vi "Build_Asylum_SetSTFC.vi"(6 "trigger":cluster{"Value":dbl, "greaterOrLesser":dbl}, 7 "eventString":string, 8 "error in (no error)":errorcluster, 9 "inChannelString":string, 10 "time":dbl, 11 "z":cluster{"Start":dbl, "End":dbl}) -> (0 "error out":errorcluster, 3 "Command":string)   [LabVIEW 2020]
panel:
  in  "callback":string
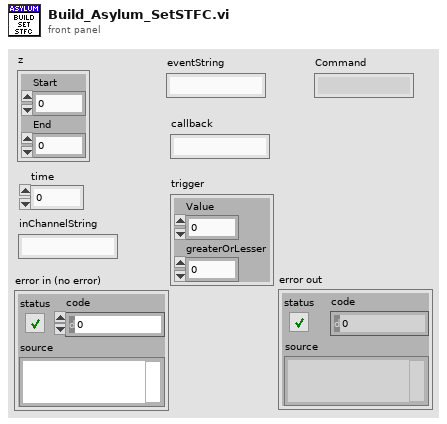
[diagram p1: front panel]
types:
  T1 = cluster{"Value":string, "greaterOrLesser":string}
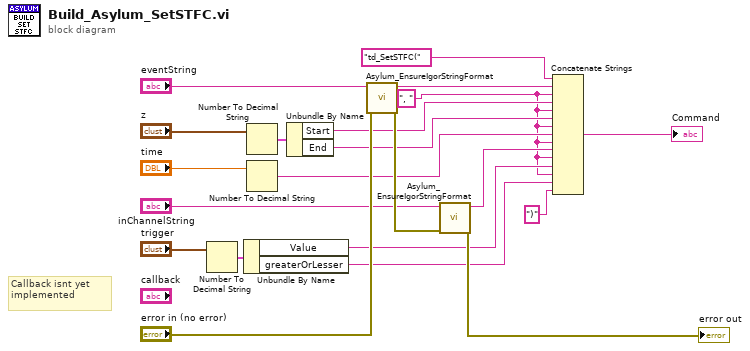
[diagram p0: block diagram]
diagram:
  w3 = ", " ("string")
  # "Callback isnt yet implemented"
  n1 = Number To Decimal String(number="trigger") -> (decimal integer string=w12:T1)  [unwired: 1 in]
  n2 = Unbundle By Name(w12) -> ("Value"=w5:string, "greaterOrLesser"=w4:string)
  n3 = Number To Decimal String(number="z") -> (decimal integer string=w13:cluster{"Start":string, "End":string})  [unwired: 1 in]
  n4 = Number To Decimal String(number="time") -> (decimal integer string=w7:string)  [unwired: 1 in]
  n5 = Unbundle By Name(w13) -> ("Start"=w9:string, "End"=w8:string)
  n6 = call "Asylum_EnsureIgorStringFormat.vi"("error in (no error)"="error in (no error)", "Value"="eventString") -> ("error out"=w21:errorcluster, "Value"=w16:string)  [unwired: 8 in]
  n7 = call "Asylum_EnsureIgorStringFormat.vi"("error in (no error)"=w21, "Value"="inChannelString") -> ("error out"=→"error out":errorcluster, "Value"=w6:string)  [unwired: 8 in]
  n8 = Concatenate Strings("td_SetSTFC(" ("string"), w16, w3, w9, w3, w8, w3, w7, w3, w6, w3, w5, w3, w4, ")" ("string")) -> (→"Command":string)
